vi "Available SPI.vi"(8 "error in (no error)":errorcluster, 11 "VisaComms in":refnum<class "VisaComms.lvclass">) -> (0 "error out":errorcluster, 2 "Available SPI":T1[](array[typedef]), 3 "VisaComms out":refnum<class "VisaComms.lvclass">)   [LabVIEW 2020, in "CTI.lvlib" / "VisaComms.lvclass"]
uses:
  VisaComms.lvclass
  Available SPI.ctl
  SPI Number.ctl
  GPIO Number.ctl
  VisaComms.lvclass/VisaComms.ctl
  CTI.lvlib
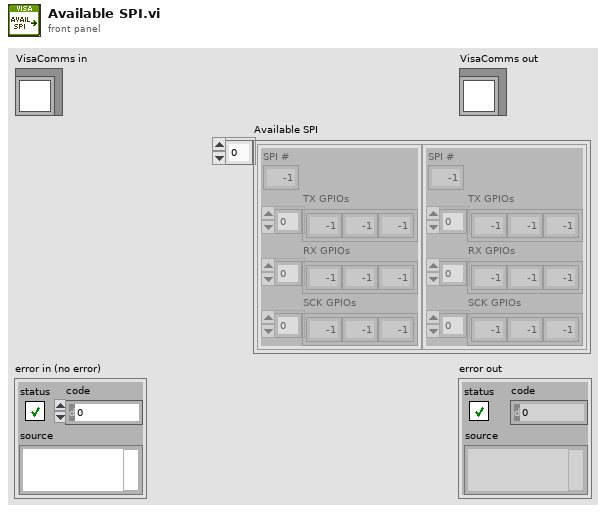
[diagram p1: front panel]
types:
  T1 = typedef "CTI.lvlib/Available SPI.ctl" = cluster{"SPI #":T2, "TX GPIOs":T3[], "RX GPIOs":T3[], "SCK GPIOs":T3[]}
  T2 = typedef "CTI.lvlib/SPI Number.ctl" = i8
  T3 = typedef "CTI.lvlib/GPIO Number.ctl" = i8
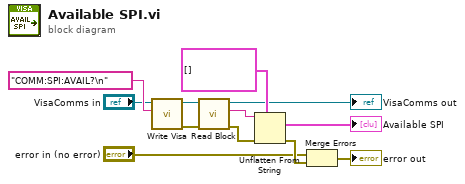
[diagram p0: block diagram]
diagram:
  n1 = call "Write Visa.vi"("write buffer"="COMM:SPI:AVAIL?\n", "VisaComms in"="VisaComms in") -> ("error out"=w9:errorcluster, "VisaComms out"=w10:refnum<class "VisaComms.lvclass">)  [unwired: 7 in, 1 out]
  n2 = call "Read Block.vi"("error in (no error)"=w9, "VisaComms in"=w10) -> ("error out"=w12:errorcluster, "Block"=w8:string, "VisaComms out"=→"VisaComms out":refnum<class "VisaComms.lvclass">)  [unwired: 7 in]
  n3 = Unflatten From String(type=T1[] [] ("Available SPI"), binary string=w8, error in (no error)=w12) -> (value=→"Available SPI":T1[], error out=w7:errorcluster)  [unwired: 2 in, 1 out]
  n4 = Merge Errors("error in (no error)", w7) -> (→"error out":errorcluster)
